vi "Library Name.vi"() -> (3 "library name":string="Memory Manager.lvlib")   [LabVIEW 2017, in "Memory Manager.lvlib"]
doc: "A set of block diagram constants used throughout this library."
uses:
  Memory Manager.lvlib
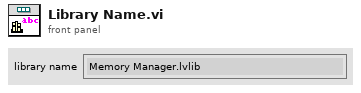
[diagram p1: front panel]
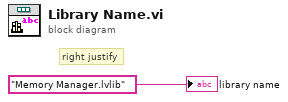
[diagram p0: block diagram]
diagram:
  # "right justify"
  "library name" <- "Memory Manager.lvlib"
